vi "GetDt.vi"(11 "props in":T1[](array[typedef])) -> (1 "found":bool, 2 "Dt":dbl, 3 "key value pairs out":T1[](array[typedef]))   [LabVIEW 2017, in "McsaStartupAnalysis.lvlib"]
uses:
  <vilib>/addons/InsightCM/Devices/Shared/Mcsa/McsaStartupAnalysis/McsaStartupAnalysis.lvlib
  <vilib>/addons/InsightCM/MessageBus/Base/controls/KeyValuePair.ctl
  <vilib>/addons/InsightCM/Utilities/PropertyHelpers/PropertyHelpers.lvlib
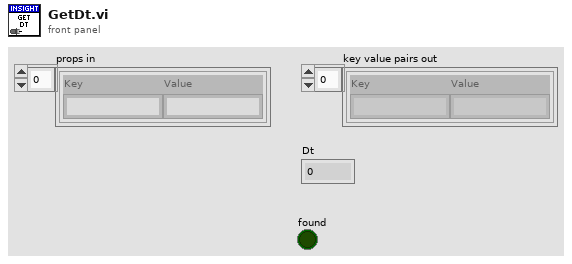
[diagram p1: front panel]
types:
  T1 = typedef "KeyValuePair.ctl" = cluster{"Key":string, "Value":string}
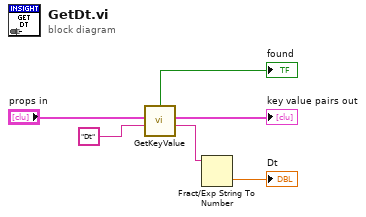
[diagram p0: block diagram]
diagram:
  n1 = call <vilib>:"GetKeyValue.vi"("key"="Dt", "key value pairs"="props in") -> ("value"=w6:string, "key value pairs out"=→"key value pairs out":T1[], "found"=→"found":bool)  [unwired: 7 in]
  n2 = Fract/Exp String To Number(string=w6) -> (number=→"Dt":dbl)  [unwired: 3 in, 1 out]
